vi "main001.vi"() -> ()   [LabVIEW 2019]
uses:
  <vilib>/DAQmx/write.llb/DAQmx Write (Analog DBL 1Chan 1Samp).vi
  <vilib>/DAQmx/miscellaneous.llb/DAQmx Fill In Error Info.vi
  <vilib>/DAQmx/create/channels.llb/DAQmx Create Channel (AO-Voltage-Basic).vi
  libs/Newport ESP301/Newport ESP301.lvlib
panel:
  out "x*y":dbl
  in  "physical channels":tag="Dev3/ao1"
  out "DAC error":errorcluster
  out "ESP error":errorcluster
  out "run?":bool
  in  "thresh":dbl
  in  "set_vel":bool
  in  "velocity [fs/s]":dbl
  in  "vel_mm":dbl caption="velocity [mm/s]"
  out "meas. velocity":dbl
  in  "stop":bool
  out "output voltage":dbl
  in  "start":bool
  in  "go2p1":bool
  out "position [fs]":dbl
  out "position [mm]":dbl
  in  "p2 [mm]":dbl
  in  "p1 [mm]":dbl
  in  "interpolate output":bool
  in  "t2 [fs]":dbl
  in  "t1 [fs]":dbl
  in  "t0 [mm]":dbl
  in  "Axis (1)":i32=1 min=1 max=3
  in  "Serial Link (RS232)":enum16{"RS232", "USB"}(ring)=enum."USB"
  in  "VISA resource name":refnum<visa-resource-name>="COM8"
  in  "main_close":bool
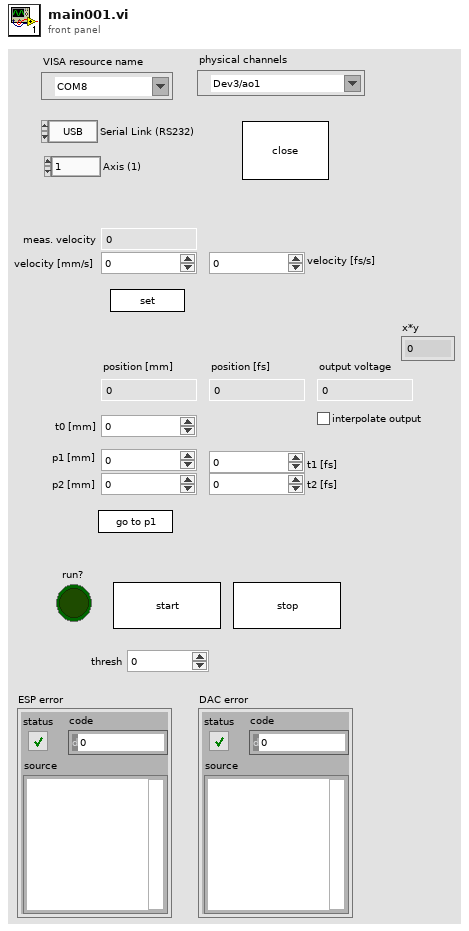
[diagram p1: front panel]
types:
  T1 = cluster{"dev1_data":refnum<queue>, "dev2_data":refnum<queue>}
  T2 = cluster{"dev1_cmd":refnum<queue>, "dev2_cmd":refnum<queue>}
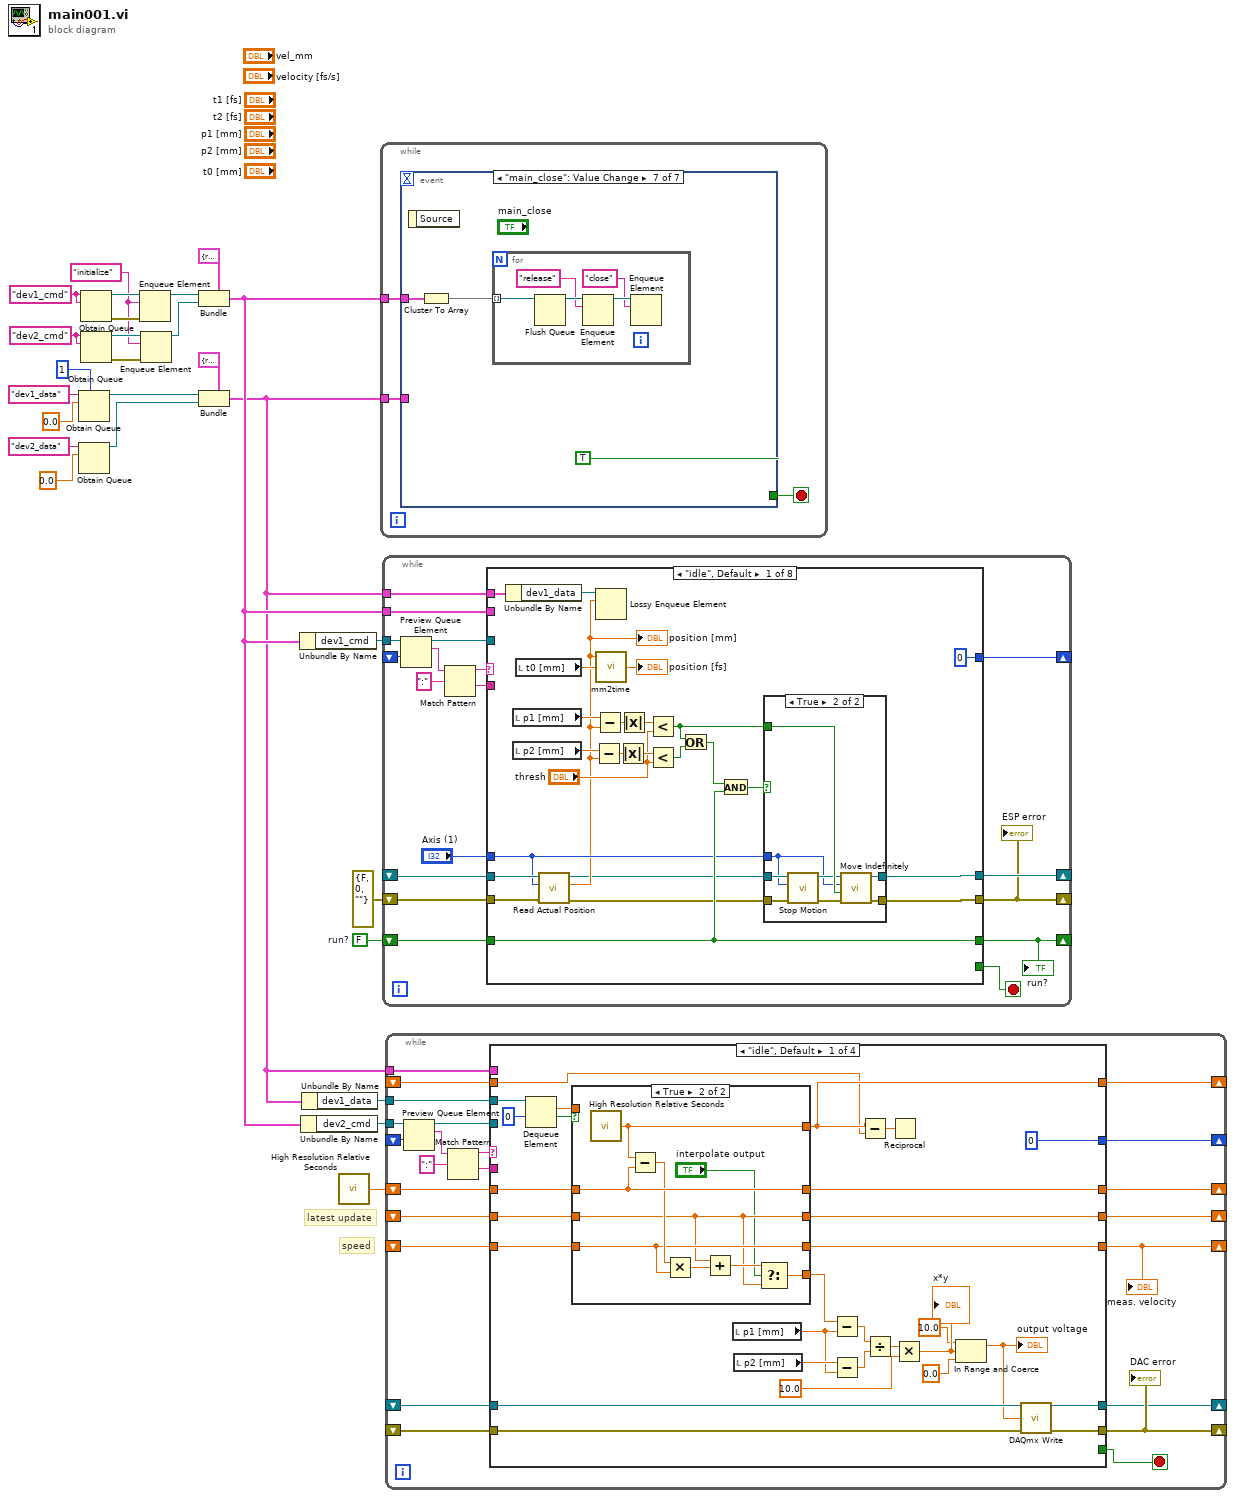
[diagram p0: block diagram]
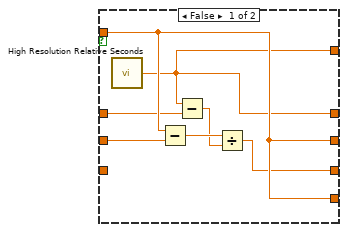
[diagram p2: hidden frame]
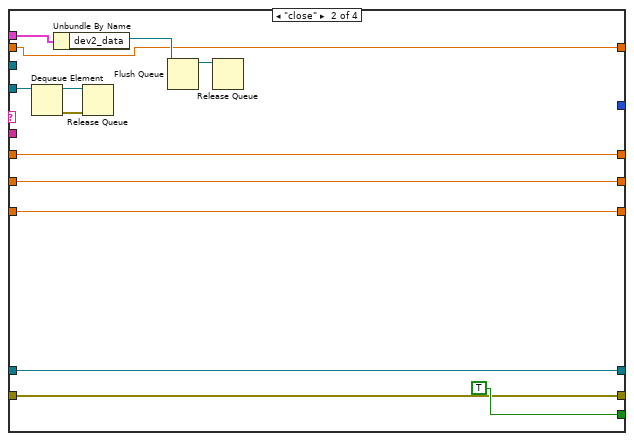
[diagram p3: hidden frame]
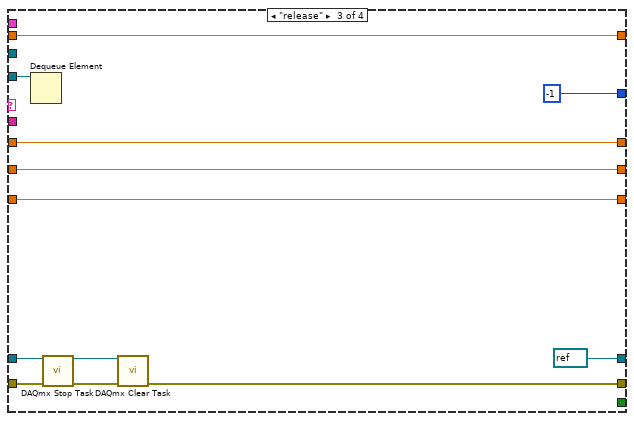
[diagram p4: hidden frame]
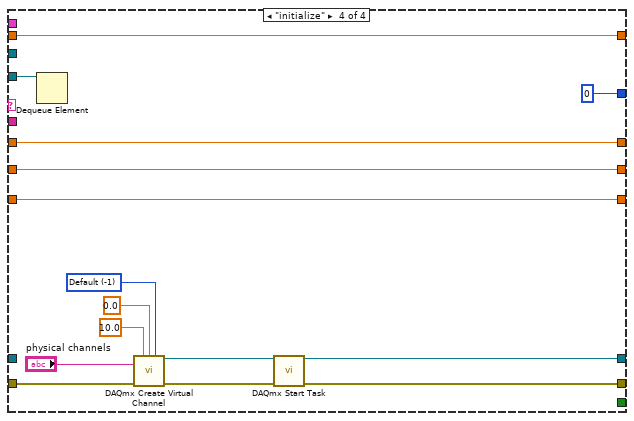
[diagram p5: hidden frame]
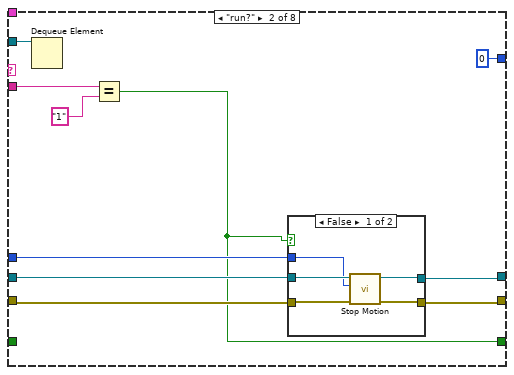
[diagram p7: hidden frame]
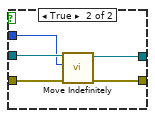
[diagram p8: hidden frame]
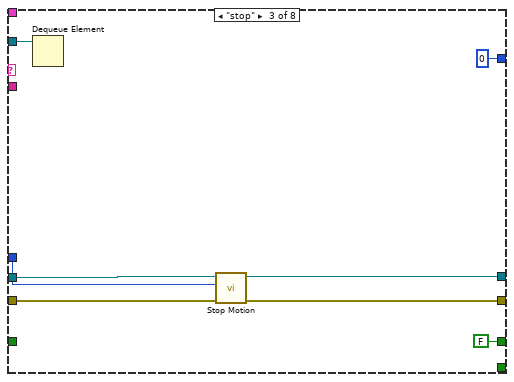
[diagram p9: hidden frame]
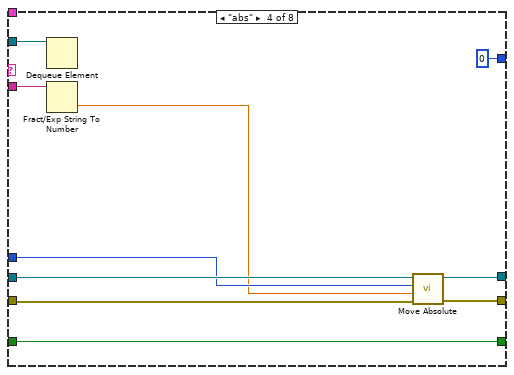
[diagram p10: hidden frame]
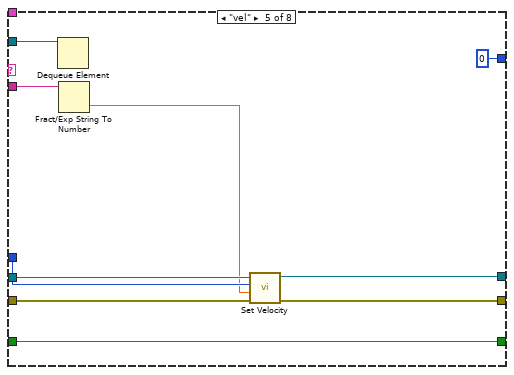
[diagram p11: hidden frame]
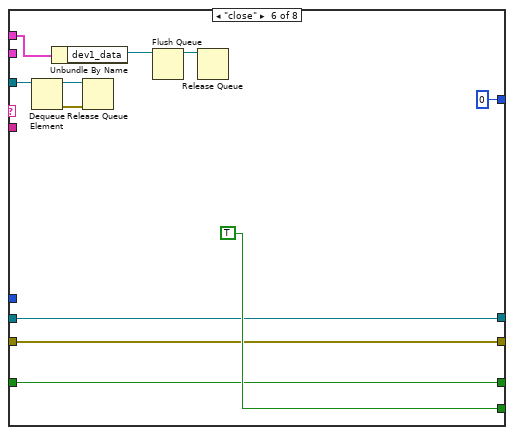
[diagram p12: hidden frame]
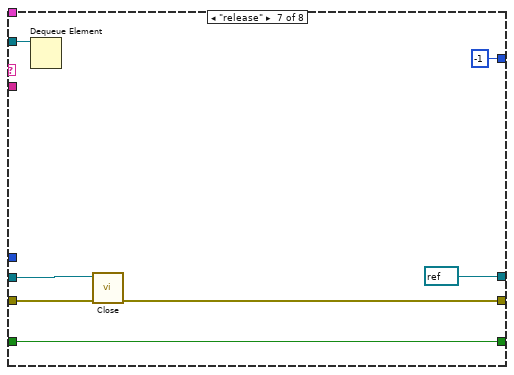
[diagram p13: hidden frame]
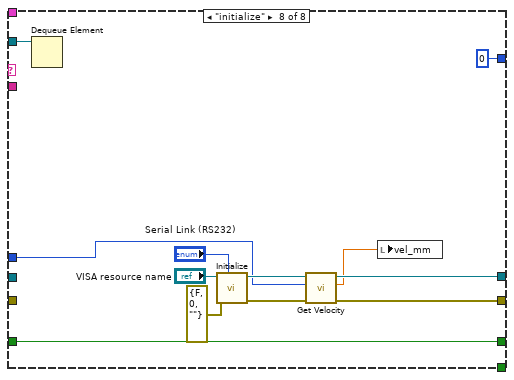
[diagram p14: hidden frame]
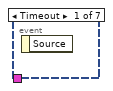
[diagram p15: hidden frame]
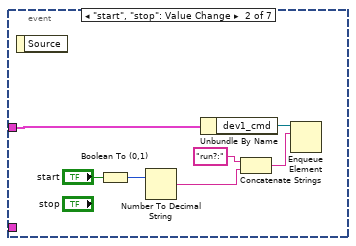
[diagram p16: hidden frame]
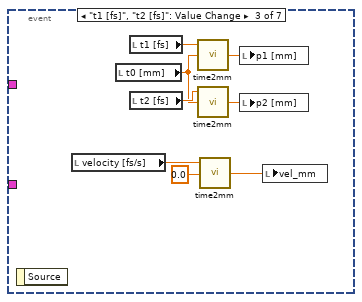
[diagram p17: hidden frame]
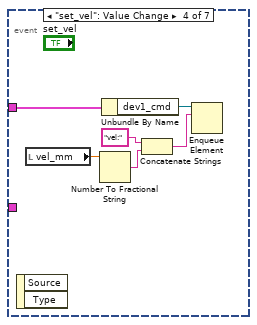
[diagram p18: hidden frame]
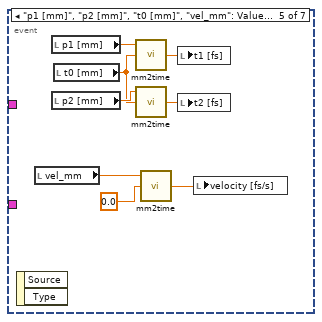
[diagram p19: hidden frame]
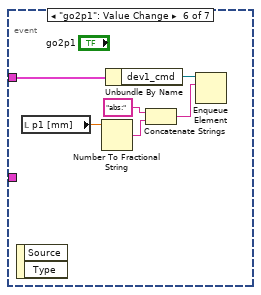
[diagram p20: hidden frame]
diagram:
  w3 = FALSE  # run?
  w14 = "dev2_cmd" ("name (unnamed)")
  w20 = "initialize" ("element")
  w15 = "dev1_cmd" ("name (unnamed)")
  # "speed"
  # "latest update"
  n1 = Obtain Queue(max queue size (-1, unlimited)=1, name (unnamed)="dev1_data", element data type=0.0) -> (queue out=w11:refnum<queue>)  [unwired: 2 in, 2 out]
  n2 = Obtain Queue(name (unnamed)="dev2_data", element data type=0.0) -> (queue out=w10:refnum<queue>)  [unwired: 3 in, 2 out]
  n3 = Obtain Queue(name (unnamed)=w15, element data type=w15) -> (queue out=w26:refnum<queue>, error out=w25:errorcluster)  [unwired: 3 in, 1 out]
  n4 = Obtain Queue(name (unnamed)=w14, element data type=w14) -> (queue out=w21:refnum<queue>, error out=w22:errorcluster)  [unwired: 3 in, 1 out]
  n5 = Enqueue Element(queue=w26, element=w20, error in (no error)=w25) -> (queue out=w23:refnum<queue>)  [unwired: 1 in, 2 out]
  n6 = Enqueue Element(queue=w21, element=w20, error in (no error)=w22) -> (queue out=w19:refnum<queue>)  [unwired: 1 in, 2 out]
  n7 = Bundle(cluster=T2 {"dev1_cmd"=refnum, "dev2_cmd"=refnum}, "dev1_cmd"=w23, "dev2_cmd"=w19) -> (w7:T2)
  n8 = Bundle(cluster=T1 {"dev1_data"=refnum, "dev2_data"=refnum}, "dev1_data"=w11, "dev2_data"=w10) -> (w1:T1)
  n9 = Unbundle By Name(w7) -> ("dev1_cmd"=w16:refnum<queue>)
  n10 = Unbundle By Name(w7) -> ("dev2_cmd"=w6:refnum<queue>)
  n11 = Unbundle By Name(w1) -> ("dev1_data"=w5:refnum<queue>)
  n12 = call <vilib>:"High Resolution Relative Seconds.vi"() -> ("relative seconds"=w4:dbl)
  n13 = while {
    tunnel: w7 -> [w29]
    tunnel: w1 -> [w28]
    stop <- w27 stop-if-true
    n14 = event shown="[6] \"main_close\": Value Change" {
      selector: _ -> [_ _ _ _ _ _ _]
      dyn-events: _ -> [_ _ _ _ _ _ _]
      timeout: _ -> [_ _ _ _ _ _ _]
      tunnel: w29 -> [_ w33 _ w46 _ w64 w67]
      tunnel: w28 -> [_ _ _ _ _ _ _]
      tunnel: [_ _ _ _ _ _ TRUE] -> w27
      event Timeout {
        n15 = event-data() -> ()  [unwired: 1 in, 1 out]
      }
      event "start", "stop": Value Change {
        n16 = event-data() -> ()  [unwired: 1 in, 1 out]
        n17 = Boolean To (0,1)(Boolean="start") -> (0, 1=w31:i16)
        n18 = Number To Decimal String(number=w31) -> (decimal integer string=w30:string)  [unwired: 1 in]
        n19 = Unbundle By Name(w33) -> ("dev1_cmd"=w36:refnum<queue>)
        n20 = Concatenate Strings("run?:" ("string"), w30) -> (w35:string)
        n21 = Enqueue Element(queue=w36, element=w35) -> ()  [unwired: 2 in, 3 out]
      }
      event "t1 [fs]", "t2 [fs]": Value Change {
        n22 = event-data() -> ()  [unwired: 1 in, 1 out]
        n23 = local read "velocity [fs/s]"() -> (w39:dbl)
        n24 = local read "t0 [mm]"() -> (w42:dbl)
        n25 = local read "t1 [fs]"() -> (w43:dbl)
        n26 = local read "t2 [fs]"() -> (w44:dbl)
        n27 = call "time2mm.vi"("Offset (mm)"=w42, "time"=w43) -> ("position (mm)"=w40:dbl)  [unwired: 1 in]
        n28 = call "time2mm.vi"("Offset (mm)"=w42, "time"=w44) -> ("position (mm)"=w41:dbl)  [unwired: 1 in]
        n29 = call "time2mm.vi"("Offset (mm)"=0.0, "time"=w39) -> ("position (mm)"=w37:dbl)  [unwired: 1 in]
        n30 = local write "p1 [mm]"(w40) -> ()
        n31 = local write "p2 [mm]"(w41) -> ()
        n32 = local write "vel_mm"(w37) -> ()
      }
      event "set_vel": Value Change {
        n33 = event-data() -> ()  [unwired: 1 in, 2 out]
        n34 = local read "vel_mm"() -> (w45:dbl)
        n35 = Number To Fractional String(number=w45) -> (F-format string=w49:string)  [unwired: 3 in]
        n36 = Unbundle By Name(w46) -> ("dev1_cmd"=w50:refnum<queue>)
        n37 = Concatenate Strings("vel:" ("string"), w49) -> (w48:string)
        n38 = Enqueue Element(queue=w50, element=w48) -> ()  [unwired: 2 in, 3 out]
      }
      event "p1 [mm]", "p2 [mm]", "t0 [mm]", "vel_mm": Value Change {
        n39 = event-data() -> ()  [unwired: 1 in, 2 out]
        n40 = local read "vel_mm"() -> (w53:dbl)
        n41 = local read "p1 [mm]"() -> (w57:dbl)
        n42 = local read "p2 [mm]"() -> (w58:dbl)
        n43 = local read "t0 [mm]"() -> (w56:dbl)
        n44 = call "mm2time.vi"("Offset (mm)"=w56, "distance (mm)"=w57) -> ("time in fs"=w54:dbl)  [unwired: 1 in]
        n45 = call "mm2time.vi"("Offset (mm)"=w56, "distance (mm)"=w58) -> ("time in fs"=w55:dbl)  [unwired: 1 in]
        n46 = call "mm2time.vi"("Offset (mm)"=0.0, "distance (mm)"=w53) -> ("time in fs"=w52:dbl)  [unwired: 1 in]
        n47 = local write "t1 [fs]"(w54) -> ()
        n48 = local write "t2 [fs]"(w55) -> ()
        n49 = local write "velocity [fs/s]"(w52) -> ()
      }
      event "go2p1": Value Change {
        n50 = event-data() -> ()  [unwired: 1 in, 2 out]
        n51 = local read "p1 [mm]"() -> (w59:dbl)
        n52 = Number To Fractional String(number=w59) -> (F-format string=w62:string)  [unwired: 3 in]
        n53 = Unbundle By Name(w64) -> ("dev1_cmd"=w63:refnum<queue>)
        n54 = Concatenate Strings("abs:" ("string"), w62) -> (w60:string)
        n55 = Enqueue Element(queue=w63, element=w60) -> ()  [unwired: 2 in, 3 out]
      }
      event "main_close": Value Change {
        n56 = event-data() -> ()  [unwired: 1 in, 1 out]
        n57 = Cluster To Array(cluster=w67) -> (array=w66:refnum<queue>[])
        n58 = for {
          tunnel: w66 -> [w72] mode=indexing
          n59 = Flush Queue(queue=w72) -> (queue out=w71:refnum<queue>)  [unwired: 1 in, 2 out]
          n60 = Enqueue Element(queue=w71, element="release") -> (queue out=w69:refnum<queue>)  [unwired: 2 in, 2 out]
          n61 = Enqueue Element(queue=w69, element="close") -> ()  [unwired: 2 in, 3 out]
        }
      }
    }
  }
  n62 = while {
    tunnel: w7 -> [w85]
    tunnel: w16 -> [w90]
    tunnel: w1 -> [w82]
    shift-right: [w80] -> _
    shift-left: _ -> [w81]
    shift-right: [w79] -> _
    shift-left: _ -> [w76]
    shift-right: [w78] -> _
    shift-left: errorcluster {"status"=FALSE, "code"=0, "source"=""} ("error out") -> [w77]
    shift-right: [w73] -> _
    shift-left: w3 -> [w74]
    stop <- w83 stop-if-true
    n63 = Preview Queue Element(queue=w90, timeout in ms (-1)=w81) -> (queue out=w84:refnum<queue>, element=w89:string)  [unwired: 1 in, 2 out]
    n64 = Match Pattern(string=w89, regular expression=":") -> (before substring=w87:string, after substring=w86:string)  [unwired: 1 in, 2 out]
    n65 = case shown="\"idle\", Default" w87 {
      tunnel: w86 -> [_ w135 _ w162 w168 _ _ _]
      tunnel: w85 -> [_ _ _ _ _ _ _ _]
      tunnel: w84 -> [_ w133 w146 w163 w166 w184 w190 w199]
      tunnel: [_ _ _ _ _ TRUE _ _] -> w83
      tunnel: w82 -> [w114 _ _ _ _ w176 _ _]
      tunnel: [0 0 0 0 0 0 -1 0] -> w80
      tunnel: [w101 w130 w151 w159 w173 w180 refnum<visa-resource-name> refnum ("VISA resource name out") w195] -> w79
      tunnel: [w100 w129 w150 w158 w172 w179 w187 w194] -> w78
      tunnel: w77 -> [w94 w127 w152 w160 w171 w179 w188 _]
      tunnel: w76 -> [w96 w128 w153 w161 w170 w180 w189 _]
      tunnel: "Axis (1)" -> [w95 w131 w149 w157 w169 _ _ w196]
      tunnel: w74 -> [w102 _ _ w154 w164 w177 w185 w200]
      tunnel: [w102 w126 FALSE ("run?") w154 w164 w177 w185 w200] -> w73
      frame "idle", Default {
        n66 = Unbundle By Name(w114) -> ("dev1_data"=w113:refnum<queue>)
        n67 = local read "p1 [mm]"() -> (w110:dbl)
        n68 = local read "p2 [mm]"() -> (w105:dbl)
        n69 = local read "t0 [mm]"() -> (w112:dbl)
        n70 = call "Read Actual Position.vi"("error in (no error)"=w94, "Axis (1)"=w95, "VISA resource name"=w96) -> ("error out"=w93:errorcluster, "Position (units)"=w92:dbl, "VISA resource name out"=w91:refnum<visa-resource-name>)  [unwired: 2 in]
        "position [mm]" <- w92
        n71 = Subtract(x=w105, y=w92) -> (x-y=w106:dbl)
        n72 = Subtract(x=w110, y=w92) -> (x-y=w109:dbl)
        n73 = Lossy Enqueue Element(queue=w113, element=w92) -> ()  [unwired: 1 in, 4 out]
        n74 = call "mm2time.vi"("Offset (mm)"=w112, "distance (mm)"=w92) -> ("time in fs"=→"position [fs]":dbl)  [unwired: 1 in]
        n75 = Absolute Value(x=w106) -> (abs(x)=w107:dbl)
        n76 = Absolute Value(x=w109) -> (abs(x)=w108:dbl)
        n77 = Less?(x=w108, y="thresh") -> (x < y?=w99:bool)
        n78 = Less?(x=w107, y="thresh") -> (x < y?=w98:bool)
        n79 = Or(x=w99, y=w98) -> (x .or. y?=w103:bool)
        n80 = And(x=w103, y=w102) -> (x .and. y?=w97:bool)
        n81 = case shown="True" w97 {
          tunnel: w91 -> [w117 w122]
          tunnel: w93 -> [w116 w121]
          tunnel: [w117 w125] -> w101
          tunnel: [w116 w124] -> w100
          tunnel: w99 -> [_ w123]
          tunnel: w95 -> [_ w118]
          frame False {
          }
          frame True {
            n82 = call "Stop Motion.vi"("error in (no error)"=w121, "Axis (1)"=w118, "VISA resource name"=w122) -> ("error out"=w119:errorcluster, "VISA resource name out"=w120:refnum<visa-resource-name>)  [unwired: 3 in]
            n83 = call "Move Indefinitely.vi"("error in (no error)"=w119, "Move Direction (+)"=w123, "Axis (1)"=w118, "VISA resource name"=w120) -> ("error out"=w124:errorcluster, "VISA resource name out"=w125:refnum<visa-resource-name>)  [unwired: 2 in]
          }
        }
      }
      frame "run?" {
        n84 = Dequeue Element(queue=w133) -> ()  [unwired: 2 in, 4 out]
        n85 = Equal?(x=w135, y="1") -> (x = y?=w126:bool)
        n86 = case shown="False" w126 {
          tunnel: w128 -> [w140 w145]
          tunnel: w127 -> [w137 w144]
          tunnel: w131 -> [w136 w143]
          tunnel: [w139 w142] -> w130
          tunnel: [w138 w141] -> w129
          frame False {
            n87 = call "Stop Motion.vi"("error in (no error)"=w137, "Axis (1)"=w136, "VISA resource name"=w140) -> ("error out"=w138:errorcluster, "VISA resource name out"=w139:refnum<visa-resource-name>)  [unwired: 3 in]
          }
          frame True {
            n88 = call "Move Indefinitely.vi"("error in (no error)"=w144, "Axis (1)"=w143, "VISA resource name"=w145) -> ("error out"=w141:errorcluster, "VISA resource name out"=w142:refnum<visa-resource-name>)  [unwired: 3 in]
          }
        }
      }
      frame "stop" {
        n89 = Dequeue Element(queue=w146) -> ()  [unwired: 2 in, 4 out]
        n90 = call "Stop Motion.vi"("error in (no error)"=w152, "Axis (1)"=w149, "VISA resource name"=w153) -> ("error out"=w150:errorcluster, "VISA resource name out"=w151:refnum<visa-resource-name>)  [unwired: 3 in]
      }
      frame "abs" {
        n91 = Dequeue Element(queue=w163) -> ()  [unwired: 2 in, 4 out]
        n92 = Fract/Exp String To Number(string=w162) -> (number=w156:dbl)  [unwired: 3 in, 1 out]
        n93 = call "Move Absolute.vi"("error in (no error)"=w160, "Position (0 units)"=w156, "Axis (1)"=w157, "VISA resource name"=w161) -> ("error out"=w158:errorcluster, "VISA resource name out"=w159:refnum<visa-resource-name>)  [unwired: 2 in]
      }
      frame "vel" {
        n94 = Dequeue Element(queue=w166) -> ()  [unwired: 2 in, 4 out]
        n95 = Fract/Exp String To Number(string=w168) -> (number=w167:dbl)  [unwired: 3 in, 1 out]
        n96 = call "Set Velocity.vi"("error in (no error)"=w171, "Velocity (units/s)"=w167, "Axis (1)"=w169, "VISA resource name"=w170) -> ("error out"=w172:errorcluster, "VISA resource name out"=w173:refnum<visa-resource-name>)  [unwired: 2 in]
      }
      frame "close" {
        n97 = Dequeue Element(queue=w184) -> (queue out=w183:refnum<queue>, error out=w182:errorcluster)  [unwired: 2 in, 2 out]
        n98 = Unbundle By Name(w176) -> ("dev1_data"=w174:refnum<queue>)
        n99 = Release Queue(queue=w183, error in (no error)=w182) -> ()  [unwired: 1 in, 3 out]
        n100 = Flush Queue(queue=w174) -> (queue out=w175:refnum<queue>)  [unwired: 1 in, 2 out]
        n101 = Release Queue(queue=w175) -> ()  [unwired: 2 in, 3 out]
      }
      frame "release" {
        n102 = Dequeue Element(queue=w190) -> ()  [unwired: 2 in, 4 out]
        n103 = call "Close.vi"("error in (no error)"=w188, "VISA resource name"=w189) -> ("error out"=w187:errorcluster)  [unwired: 9 in]
      }
      frame "initialize" {
        n104 = Dequeue Element(queue=w199) -> ()  [unwired: 2 in, 4 out]
        n105 = call "Initialize.vi"("VISA resource name"="VISA resource name", "error in (no error)"=errorcluster {"status"=FALSE, "code"=0, "source"=""}, "Serial Link (RS232)"="Serial Link (RS232)") -> ("VISA resource name out"=w198:refnum<visa-resource-name>, "error out"=w197:errorcluster)  [unwired: 6 in]
        n106 = call "Get Velocity.vi"("error in (no error)"=w197, "Axis (1)"=w196, "VISA resource name"=w198) -> ("error out"=w194:errorcluster, "Velocity (units/s)"=w193:dbl, "VISA resource name out"=w195:refnum<visa-resource-name>)  [unwired: 2 in]
        n107 = local write "vel_mm"(w193) -> ()
      }
    }
    "run?" <- w73
    "ESP error" <- w78
  }
  n108 = while {
    shift-right: [w219] -> _
    shift-left: _ -> [w220]
    shift-right: [w218] -> _
    shift-left: _ -> [w217]
    tunnel: w6 -> [w216]
    shift-right: [w215] -> _
    shift-left: _ -> [w214]
    tunnel: w5 -> [w213]
    shift-right: [w212] -> _
    shift-left: _ -> [w209]
    shift-right: [w211] -> _
    shift-left: w4 -> [w210]
    shift-right: [w204] -> _
    shift-left: _ -> [w208]
    tunnel: w1 -> [w207]
    shift-right: [w206] -> _
    shift-left: _ -> [w205]
    stop <- w221 stop-if-true
    n109 = Preview Queue Element(queue=w216, timeout in ms (-1)=w220) -> (queue out=w222:refnum<queue>, element=w226:string)  [unwired: 1 in, 2 out]
    n110 = Match Pattern(string=w226, regular expression=":") -> (before substring=w224:string, after substring=w223:string)  [unwired: 1 in, 2 out]
    n111 = case shown="\"idle\", Default" w224 {
      tunnel: w223 -> [_ _ _ _]
      tunnel: w222 -> [_ w284 w295 w303]
      tunnel: [_ TRUE _ _] -> w221
      tunnel: [0 _ -1 0] -> w219
      tunnel: [w251 w280 w294 w304] -> w218
      tunnel: w217 -> [w249 w280 w291 w311]
      tunnel: [w252 w279 refnum<k21> refnum ("task out") w305] -> w215
      tunnel: w214 -> [w250 w279 w292 _]
      tunnel: w213 -> [w253 _ _ _]
      tunnel: [w247 w277 w287 w300] -> w212
      tunnel: [w246 w278 w288 w301] -> w211
      tunnel: w210 -> [w244 w278 w288 w301]
      tunnel: w209 -> [w245 w277 w287 w300]
      tunnel: [w243 w276 w286 w299] -> w204
      tunnel: w208 -> [w242 w276 w286 w299]
      tunnel: w207 -> [_ w273 _ _]
      tunnel: [w229 w272 w285 w297] -> w206
      tunnel: w205 -> [w228 w272 w285 w297]
      frame "idle", Default {
        n112 = Dequeue Element(queue=w253, timeout in ms (-1)=0) -> (element=w248:dbl, timed out?=w230:bool)  [unwired: 1 in, 2 out]
        n113 = case shown="True" w230 {
          tunnel: w248 -> [w262 _]
          tunnel: [w262 w264] -> w241
          tunnel: [w262 w266] -> w247
          tunnel: [w256 w271] -> w246
          tunnel: w245 -> [w261 w266]
          tunnel: w244 -> [w260 w271]
          tunnel: [w257 w268] -> w243
          tunnel: w242 -> [_ w268]
          tunnel: [w256 w263] -> w229
          frame False {
            n114 = call <vilib>:"High Resolution Relative Seconds.vi"() -> ("relative seconds"=w256:dbl)
            n115 = Subtract(x=w262, y=w261) -> (x-y=w259:dbl)
            n116 = Subtract(x=w256, y=w260) -> (x-y=w258:dbl)
            n117 = Divide(x=w259, y=w258) -> (x/y=w257:dbl)
          }
          frame True {
            n118 = call <vilib>:"High Resolution Relative Seconds.vi"() -> ("relative seconds"=w263:dbl)
            n119 = Subtract(x=w263, y=w271) -> (x-y=w270:dbl)
            n120 = Multiply(x=w270, y=w268) -> (x*y=w269:dbl)
            n121 = Add(x=w266, y=w269) -> (x+y=w267:dbl)
            n122 = Select(t=w267, s="interpolate output", f=w266) -> (s? t:f=w264:dbl)
          }
        }
        n123 = local read "p1 [mm]"() -> (w239:dbl)
        n124 = local read "p2 [mm]"() -> (w240:dbl)
        n125 = Subtract(x=w241, y=w239) -> (x-y=w238:dbl)
        n126 = Subtract(x=w240, y=w239) -> (x-y=w237:dbl)
        n127 = Subtract(x=w229, y=w228) -> (x-y=w227:dbl)
        n128 = Divide(x=w238, y=w237) -> (x/y=w236:dbl)
        n129 = Reciprocal(x=w227) -> ()  [unwired: 1 out]
        n130 = Multiply(x=w236, y=10.0) -> (x*y=w234:dbl)
        "x*y" <- w234
        n131 = In Range and Coerce(upper limit=10.0, x=w234, lower limit=0.0) -> (coerced(x)=w231:dbl)  [unwired: 1 out]
        "output voltage" <- w231
        n132 = call-poly <vilib>:"DAQmx Write.vi"("task/channels in"=w250, "data"=w231, "error in"=w249) -> ("task out"=w252:refnum<k21>, "error out"=w251:errorcluster)  [unwired: 10 in, 1 out]
      }
      frame "close" {
        n133 = Dequeue Element(queue=w284) -> (queue out=w283:refnum<queue>, error out=w282:errorcluster)  [unwired: 2 in, 2 out]
        n134 = Unbundle By Name(w273) -> ("dev2_data"=w274:refnum<queue>)
        n135 = Release Queue(queue=w283, error in (no error)=w282) -> ()  [unwired: 1 in, 3 out]
        n136 = Flush Queue(queue=w274) -> (queue out=w275:refnum<queue>)  [unwired: 1 in, 2 out]
        n137 = Release Queue(queue=w275) -> ()  [unwired: 2 in, 3 out]
      }
      frame "release" {
        n138 = Dequeue Element(queue=w295) -> ()  [unwired: 2 in, 4 out]
        n139 = call <vilib>:"DAQmx Stop Task.vi"("task/channels in"=w292, "error in"=w291) -> ("task out"=w290:refnum<k21>, "error out"=w289:errorcluster)  [unwired: 12 in]
        n140 = call <vilib>:"DAQmx Clear Task.vi"("task in"=w290, "error in"=w289) -> ("error out"=w294:errorcluster)  [unwired: 13 in]
      }
      frame "initialize" {
        w308 = -1 items=["Default"=-1, "RSE"=10083, "Differential"=10106, "Pseudodifferential"=12529] ("output terminal configuration")
        n141 = Dequeue Element(queue=w303) -> ()  [unwired: 2 in, 4 out]
        n142 = call-poly <vilib>:"DAQmx Create Virtual Channel.vi"("maximum value"=10.0, "minimum value"=0.0, "output terminal configuration"=w308, "physical channels"="physical channels", "error in"=w311) -> ("task out"=w307:refnum<k21>, "error out"=w306:errorcluster)  [unwired: 9 in]
        n143 = call <vilib>:"DAQmx Start Task.vi"("task/channels in"=w307, "error in"=w306) -> ("task out"=w305:refnum<k21>, "error out"=w304:errorcluster)  [unwired: 12 in]
      }
    }
    "meas. velocity" <- w204
    "DAC error" <- w218
  }
